vi "Serial To Complex IQ Data.vi"(8 "error in (no error)":errorcluster, 10 "FFT Size":i32, 11 "Serial Data In":refnum<class "1D Array s16.lvclass">) -> (0 "error out":errorcluster, 1 "Batch Count":u64, 2 "Amount Of Samples":u64, 3 "Batched Complex Data Out":refnum<class "2D Array c32.lvclass">)   [LabVIEW 2025, in "Signal Analysis.lvlib" / "Signal Analysis.lvclass"]
uses:
  Signal Analysis.lvclass
  Signal Analysis.lvclass/Signal Analysis.ctl
  <vilib>/Natan Biesmans/G2CPU GPU and CPU HPC Toolkit/G2CPU Libraries/Arrays/1DArray/s16/1D Array s16.lvclass
  <vilib>/Natan Biesmans/G2CPU GPU and CPU HPC Toolkit/G2CPU Libraries/Arrays/Array/Array Prototype.lvclass
  a8033d75-3945-452f-b18c-39e28a7b0aba.vi
  6eb05897-42b9-4ca8-a27f-aa2d2922260c.vi
  f7af0358-a13b-4a6d-a862-4bbb6758827b.vi
  bed188cd-c5b4-4062-88ca-95769998f335.vi
  fdaa73c4-b8c4-409b-8662-37d77ce6d9f3.vi
  a4ca7f78-b574-49ca-a0de-46a0a2fe7209.vi
  <vilib>/Natan Biesmans/G2CPU GPU and CPU HPC Toolkit/G2CPU Libraries/Arrays/2DArray/c32/2D Array c32.lvclass
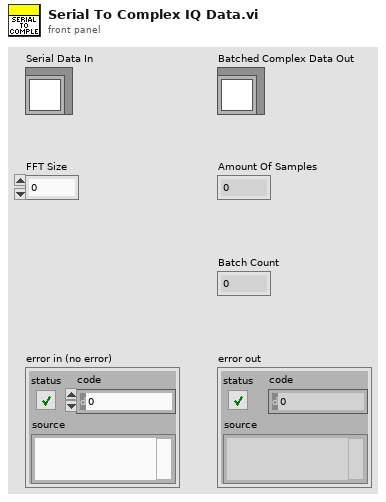
[diagram p1: front panel]
types:
  T1 = typedef "AF.lvlib/Dim4.ctl" = cluster{"Dim 0":u64, "Dim 1":u64, "Dim 2":u64, "Dim 3":u64}
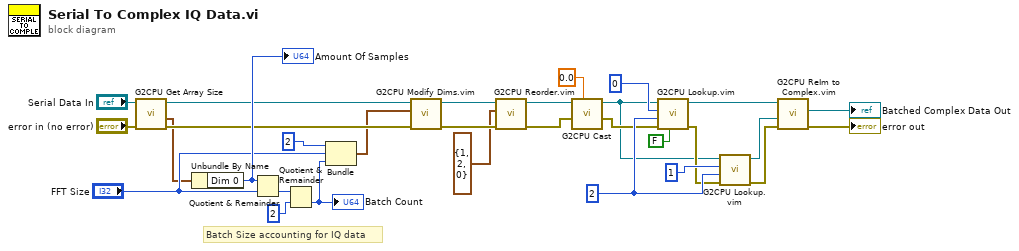
[diagram p0: block diagram]
diagram:
  w21 = 2
  # "Batch Size accounting for IQ data"
  n1 = call <vilib>:"G2CPU Get Array Size.vi"("error in (no error)"="error in (no error)", "Array in"="Serial Data In") -> ("error out"=w23:errorcluster, "Array Size"=w4:T1, "Array out"=w24:refnum<class "1D Array s16.lvclass">)  [unwired: 6 in, 1 out]
  n2 = Unbundle By Name(w4) -> ("Dim 0"=w30:u64)
  "Amount Of Samples" <- w30
  n3 = Quotient & Remainder(x=w30, y="FFT Size") -> (floor(x/y)=w27:u64)  [unwired: 1 out]
  n4 = Quotient & Remainder(x=w27, y=2) -> (floor(x/y)=w1:u64)  [unwired: 1 out]
  "Batch Count" <- w1
  n5 = Bundle(2, "FFT Size"="FFT Size", w1) -> (w5:cluster{i32, "FFT Size":i32, u64})  [unwired: 1 in]
  n6 = call "G2CPU Modify Dims.vim"("error in (no error)"=w23, "dims"=w5, "Array In"=w24) -> ("error out"=w22:errorcluster, "Array out"=w7:refnum<class "3D Array s16.lvclass">)  [unwired: 7 in]
  n7 = call "G2CPU Reorder.vim"("error in (no error)"=w22, "Dim reorder"=cluster{"Dim 0":u64, "Dim 1":u64, "Dim 2":u64} {"Dim 0"=1, "Dim 1"=2, "Dim 2"=0}, "Array In"=w7) -> ("error out"=w9:errorcluster, "Array out"=w8:refnum<class "3D Array s16.lvclass">)  [unwired: 7 in]
  n8 = call "G2CPU Cast"("Datatype Prototype"=sgl 0.0, "error in (no error)"=w9, "Array In"=w8) -> ("error out"=w15:errorcluster, "Array Out"=w12:refnum<class "3D Array f32.lvclass">)  [unwired: 7 in]
  n9 = call "G2CPU Lookup.vim"("Auto Release Array In (Enabled)"=FALSE, "error in (no error)"=w15, "dim"=w21, "Indices (1D)"=0, "Array In"=w12) -> ("error out"=w16:errorcluster, "Indexed Array"=w13:refnum<class "2D Array f32.lvclass">)  [unwired: 5 in]
  n10 = call "G2CPU Lookup.vim"("error in (no error)"=w16, "dim"=w21, "Indices (1D)"=1, "Array In"=w12) -> ("error out"=w17:errorcluster, "Indexed Array"=w14:refnum<class "2D Array f32.lvclass">)  [unwired: 6 in]
  n11 = call "G2CPU ReIm to Complex.vim"("error in (no error)"=w17, "Array Imaginary"=w14, "Array Real"=w13) -> ("error out"=→"error out":errorcluster, "Array Result"=→"Batched Complex Data Out":refnum<class "2D Array c32.lvclass">)  [unwired: 7 in]
